vi "Begin.vi"(8 "error in":errorcluster) -> (0 "error out":errorcluster)   [LabVIEW 2014]
doc: "Called before other user functions, this VI is expected to open initial I/O refnums, load in file data, and do all program initialization. Notice that the <B>error out</B> terminal is simply used for data flow. Wiring it to other structures or subVIs ensures that this VI runs first."
uses:
  <vilib>/Rock Robotics/WPI/DriverStation/WPI_DriverStationRobotMode2.ctl
  Robot Global Data.vi
  <vilib>/Rock Robotics/Network Tables/SD Write Boolean.vi
  <vilib>/Rock Robotics/Network Tables/SD Write String.vi
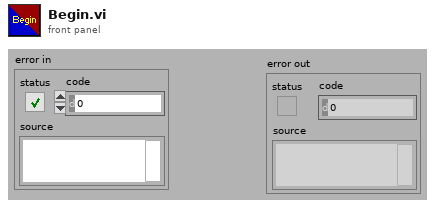
[diagram p1: front panel]
types:
  T1 = typedef "WPI_DriverStationRobotMode2.ctl" = enum16{"Autonomous Disabled", "Autonomous Enabled", "Teleop Disabled", "Teleop Enabled", "Disconnected", "Finish", "Test Disabled", "Test Enabled", "Emergency Stopped"}
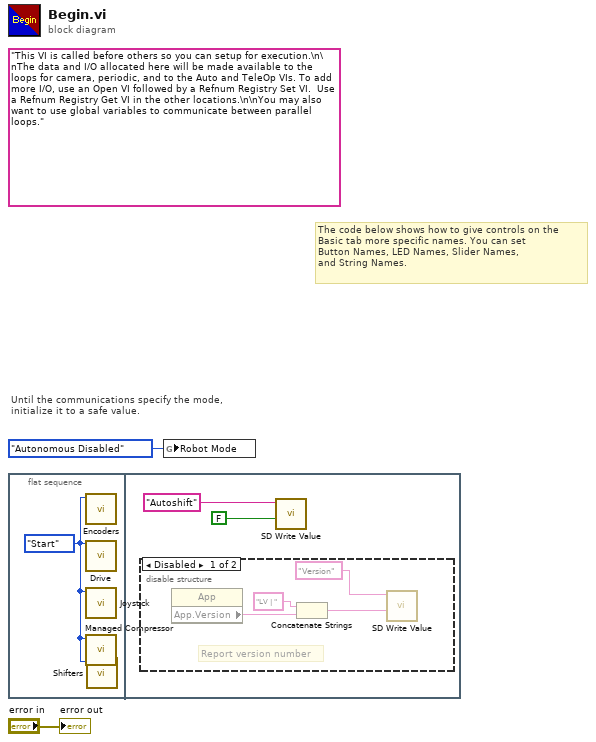
[diagram p0: block diagram]
diagram:
  (unwired) "This VI is called before others so you can setup for execution.\n\nThe data and I/O allocated here will be made available to the loops for camera, periodic, and to the Auto and TeleOp VIs. To add more I/O, use an Open VI followed by a Refnum Registry Set VI.  Use a Refnum Registry Get VI in the other locations.\n\nYou may also want to use global variables to communicate between parallel loops."
  # "The code below shows how to give controls on the\nBasic tab more specific names. You can set\nButton Names, LED Names, Slider Names,\nand String Names."
  # "Until the communications specify the mode,\ninitialize it to a safe value."
  n1 = flat-sequence {
    frame #0 {
      w3 = enum16{"Start", "Run", "End"}."Start" ("Enum")
      n2 = call "Encoders.vi"("Enum"=w3) -> ()  [unwired: 7 in, 4 out]
      n3 = call "Drive.vi"("Enum"=w3) -> ()  [unwired: 15 in]
      n4 = call "Joystick.vi"("Enum"=w3) -> ()  [unwired: 9 in, 2 out]
      n5 = call "Managed Compressor.vi"("Enum"=w3) -> ()  [unwired: 11 in]
      n6 = call "Shifters.vi"("Enum"=w3) -> ()  [unwired: 11 in]
    }
    frame #1 {
      n7 = disable-structure shown="Disabled" {
        frame Disabled {
          # "Report version number"
          n8 = property class="App"() -> ("App.Version"=w8:string)  [unwired: 2 in, 2 out]
          n9 = Concatenate Strings("LV | " ("string"), w8) -> (w6:string)
          n10 = call-poly <vilib>:"SD Write Value.vi"("String"=w6, "Name"="Version") -> ()  [unwired: 8 in, 2 out]
        }
        frame Enabled {
        }
      }
      n11 = call-poly <vilib>:"SD Write Value.vi"("Boolean"=FALSE, "Name"="Autoshift") -> ()  [unwired: 8 in, 2 out]
    }
  }
  n12 = global write "Robot Global Data.vi" "Robot Mode"(WPI_DriverStationRobotMode2."Autonomous Disabled" ("Robot Mode")) -> ()
  "error out" <- "error in"
